vi "FRCts20_Backend_Dyn_SaveXMLData.vi"(8 "error in (no error)":errorcluster, 11 "Engine_Refnums":T1) -> (0 "error out":errorcluster)   [LabVIEW 2013, in "FRCts20_Backend_DynamicLoad.lvlib"]
doc: "This VI async calls the save xml data VI"
uses:
  FRCts20_Backend_DynamicLoad.lvlib
  Dependencies/Keyed Array/KeyedArray.ctl
  Dependencies/Keyed Array/Tools_KeyedArray.lvlib
  Dependencies/AMC/_SubVIs/TypeDefs/Message.ctl
  Dependencies/AMC/AMC.lvlib
  Dependencies/AMC/_SubVIs/TypeDefs/Message Queue.ctl
  FRCts20_Backend_EngineRefnums.ctl
  FRCts20_Backend_Engine.lvlib
  <vilib>/addons/database/Connection.llb/Conn ObjectReference.ctl
  <vilib>/addons/database/NI_Database_API.lvlib
  INI_Accessor/FRCts20_Backend_INI Controller.lvclass
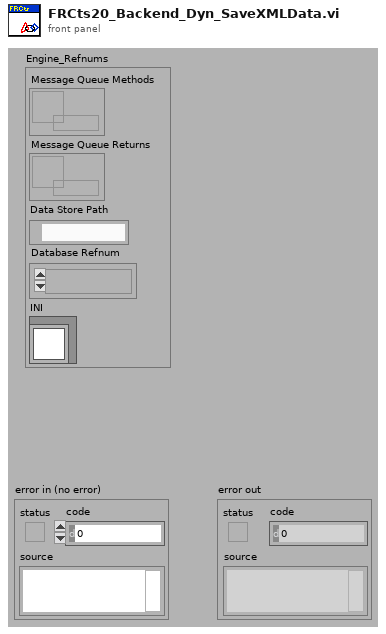
[diagram p1: front panel]
types:
  T1 = typedef "FRCts20_Backend_Engine.lvlib/FRCts20_Backend_EngineRefnums.ctl" = cluster{"Message Queue Methods":T2, "Message Queue Returns":T2, "Data Store Path":path, "Database Refnum":T3, "INI":refnum<class "FRCts20_Backend_INI Controller.lvclass">}
  T2 = typedef "AMC.lvlib/Message Queue.ctl" = refnum<queue>
  T3 = typedef "NI_Database_API.lvlib/Conn ObjectReference.ctl" = refnum<k1>
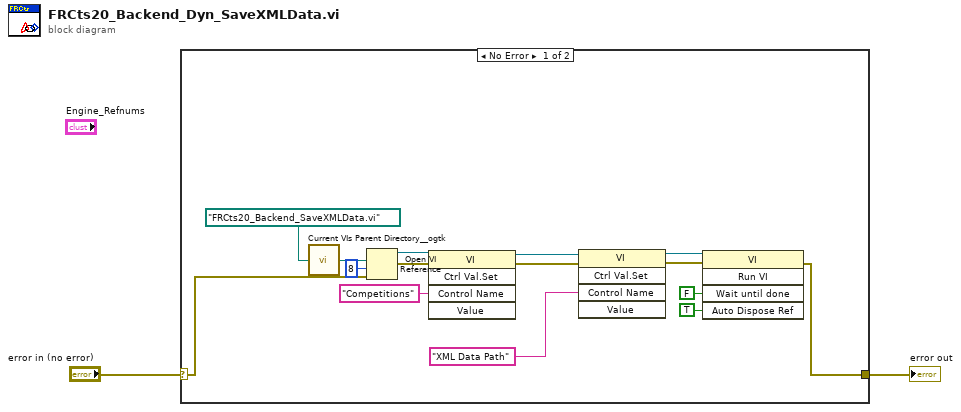
[diagram p0: block diagram]
diagram:
  n1 = case shown="No Error" "error in (no error)" {
    selector: "error in (no error)" -> [w15 w18]
    tunnel: [w4 w18] -> w1
    frame No Error {
      n2 = call "Current VIs Parent Directory__ogtk.vi"("Relative path (.)"=path "FRCts20_Backend_SaveXMLData.vi") -> ("Parent Directory (+ Relative)"=w16:path)  [unwired: 4 in]
      n3 = Open VI Reference(vi path=w16, options=8, error in (no error)=w15) -> (vi reference=w14:refnum<vi>, error out=w13:errorcluster)  [unwired: 3 in]
      n4 = invoke class="VI" method="Ctrl Val.Set"(reference=w14, error in=w13, "Control Name"="Competitions") -> (reference out=w11:refnum<vi>, error out=w10:errorcluster)  [unwired: 2 in, 3 out]
      n5 = invoke class="VI" method="Ctrl Val.Set"(reference=w11, error in=w10, "Control Name"="XML Data Path") -> (reference out=w5:refnum<vi>, error out=w6:errorcluster)  [unwired: 2 in, 3 out]
      n6 = invoke class="VI" method="Run VI"(reference=w5, error in=w6, "Wait until done"=FALSE ("Wait Until Done"), "Auto Dispose Ref"=TRUE ("Auto Dispose Reference")) -> (error out=w4:errorcluster)  [unwired: 1 in, 4 out]
    }
    frame Error {
    }
  }
  "error out" <- w1
